vi "SubVI.vi"(9 "c":dbl, 10 "b":dbl, 11 "a":dbl) -> (3 "Numeric":dbl)   [LabVIEW 2023]
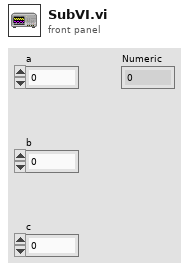
[diagram p1: front panel]
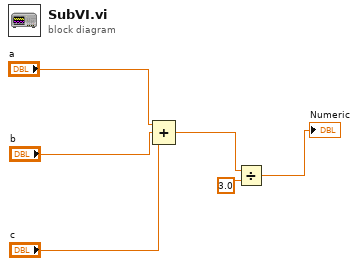
[diagram p0: block diagram]
diagram:
  n1 = Compound Arithmetic op=ADD("a", "b", "c") -> (w4:dbl)
  n2 = Divide(x=w4, y=3.0) -> (x/y=→"Numeric":dbl)
